vi "Testvi.vi"() -> ()   [LabVIEW 2015, in "Linearisierung v2.lvlib" / "Linearity verification 1065-307.lvlib"]
uses:
  Linearity verification 1065-307.lvlib
  <vilib>/Utility/miscctls.llb/LVRowAndColumnTypeDef.ctl
panel:
  out "Numerisch 2":dbl format="%#.15g"
  in  "Numerisch":dbl format="%#.15g"
  in  "OK-Schaltfläche":bool
  in  "Aktive Zelle:Aktive Zelle":T1
  in  "Stopp":bool
  out "Auswertung":string[][](table)
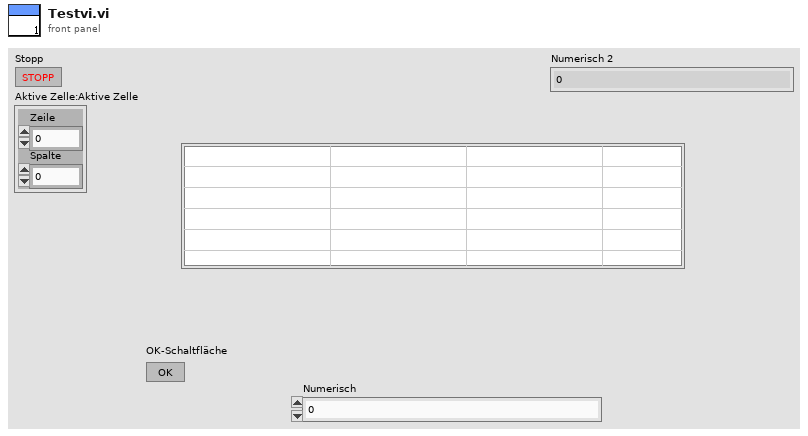
[diagram p1: front panel]
types:
  T1 = typedef "LVRowAndColumnTypeDef.ctl" = cluster{"Row":i32, "Column":i32}
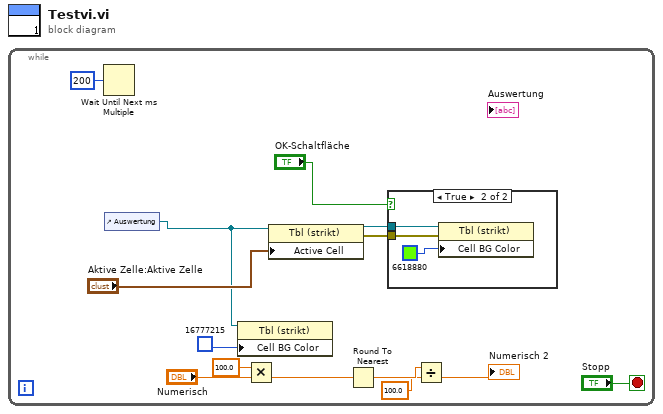
[diagram p0: block diagram]
diagram:
  n1 = while {
    stop <- "Stopp" stop-if-true
    n2 = Wait Until Next ms Multiple(millisecond multiple=u32 200 ("ms")) -> ()  [unwired: 1 out]
    n3 = control-ref of="Auswertung"() -> (w8:refnum<vi>)
    n4 = property class="Tbl (strikt)"(reference=w8, "Cell BG Color"=u32 16777215) -> ()  [unwired: 1 in, 2 out]
    n5 = Multiply(x=100.0, y="Numerisch") -> (x*y=w5:dbl)
    n6 = property class="Tbl (strikt)"(reference=w8, "Active Cell"="Aktive Zelle:Aktive Zelle") -> (reference out=w11:refnum<vi>, error out=w10:errorcluster)  [unwired: 1 in]
    n7 = Round To Nearest(number=w5) -> (nearest integer value=w2:dbl)
    n8 = case shown="True" "OK-Schaltfläche" {
      tunnel: w11 -> [_ w17]
      tunnel: w10 -> [_ w16]
      frame False {
      }
      frame True {
        n9 = property class="Tbl (strikt)"(reference=w17, error in=w16, "Cell BG Color"=u32 6618880) -> ()  [unwired: 2 out]
      }
    }
    n10 = Divide(x=w2, y=100.0) -> (x/y=→"Numerisch 2":dbl)
  }
